vi "main.vi"() -> ()   [LabVIEW 2020]
panel:
  out "x+y":dbl
  in  "y":dbl
  in  "x":dbl
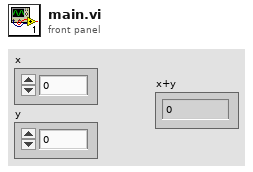
[diagram p1: front panel]
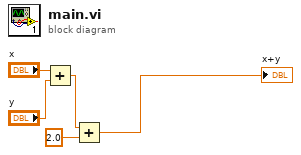
[diagram p0: block diagram]
diagram:
  n1 = Add(x="x", y="y") -> (x+y=w3:dbl)
  n2 = Add(x=w3, y=2.0) -> (x+y=→"x+y":dbl)
